vi "SR Latch.vi"(5 "Reset":bool, 9 "Value":bool) -> (3 "Latched":bool)   [LabVIEW 2018]
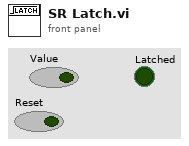
[diagram p1: front panel]
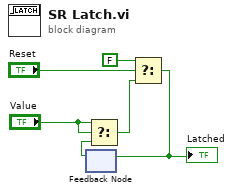
[diagram p0: block diagram]
diagram:
  n1 = feedback #1() -> (w5:bool)  [unwired: 1 in]
  n2 = Select(t="Value", s="Value", f=w5) -> (s? t:f=w3:bool)
  n3 = Select(t=FALSE, s="Reset", f=w3) -> (s? t:f=w1:bool)
  "Latched" <- w1
  n4 = feedback-in #1(w1) -> ()
